vi "LoopTime.vi"(8 "error in (no error)":errorcluster) -> (0 "error out":errorcluster, 2 "LoopTime":u32)   [LabVIEW 2013]
doc: "Use this template to build a VI to use as a subVI."
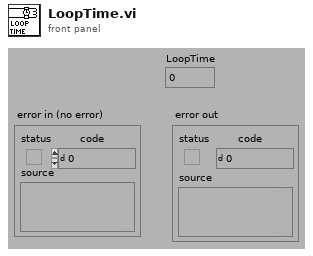
[diagram p1: front panel]
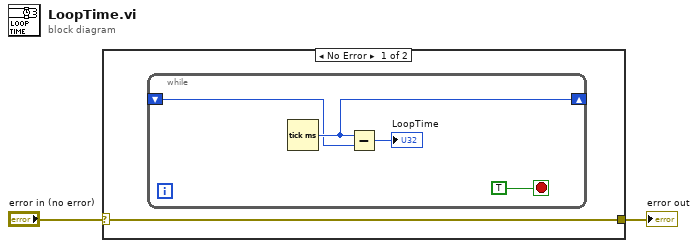
[diagram p0: block diagram]
diagram:
  n1 = case shown="No Error" "error in (no error)" {
    selector: "error in (no error)" -> [w3 w8]
    tunnel: [w3 w8] -> w1
    frame No Error {
      n2 = while {
        shift-right: [w6] -> _
        shift-left: _ -> [w5]
        stop <- TRUE stop-if-true
        n3 = Tick Count (ms)() -> (millisecond timer value=w6:u32)
        n4 = Subtract(x=w6, y=w5) -> (x-y=→"LoopTime":u32)
      }
    }
    frame Error {
    }
  }
  "error out" <- w1
